vi "mav_crc_read.vi"(11 "byte_array_in":u8[](array[numeric])=[9, 19, 1, 1, 0, 0, 0, 0, 0, 2, 3, 81, 4, 3]) -> (3 "CRC":bool)   [LabVIEW 2023]
panel:
  out "Incoming Checksum":u16
  out "Calculated Checksum":u16
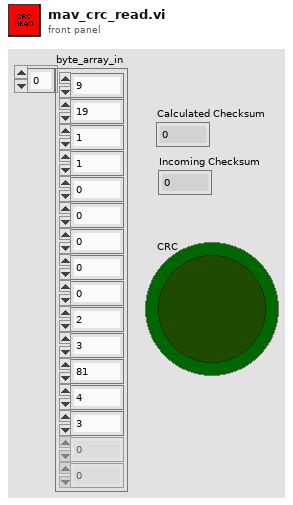
[diagram p1: front panel]
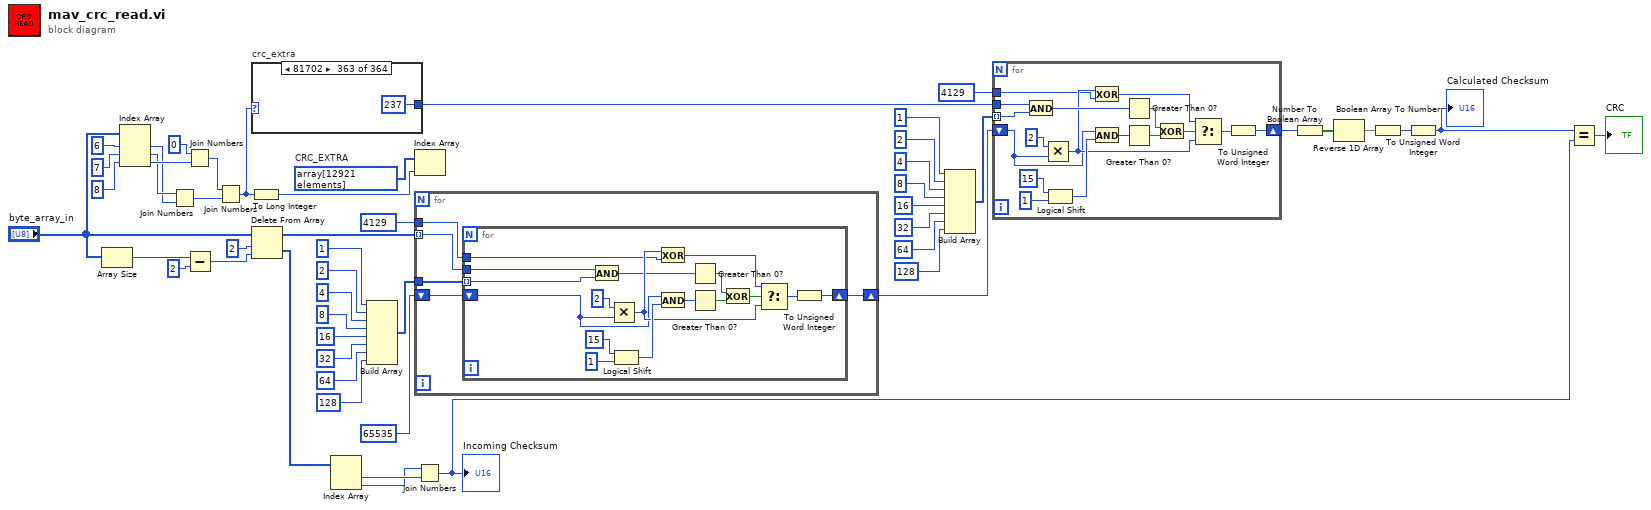
[diagram p0: block diagram]
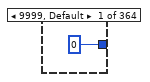
[diagram p2: hidden frame]
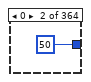
[diagram p3: hidden frame]
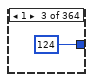
[diagram p4: hidden frame]
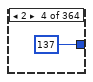
[diagram p5: hidden frame]
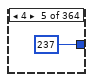
[diagram p6: hidden frame]
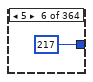
[diagram p7: hidden frame]
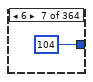
[diagram p8: hidden frame]
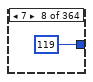
[diagram p9: hidden frame]
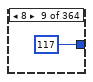
[diagram p10: hidden frame]
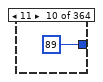
[diagram p11: hidden frame]
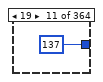
[diagram p12: hidden frame]
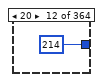
[diagram p13: hidden frame]
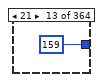
[diagram p14: hidden frame]
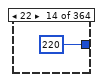
[diagram p15: hidden frame]
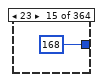
[diagram p16: hidden frame]
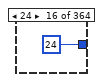
[diagram p17: hidden frame]
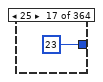
[diagram p18: hidden frame]
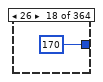
[diagram p19: hidden frame]
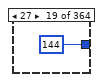
[diagram p20: hidden frame]
diagram:
  w25 = u8[] array[12921 elements]  # CRC_EXTRA
  n1 = Array Size(array="byte_array_in") -> (size(s)=w24:i32)
  n2 = Index Array(array="byte_array_in", index #1=6 ("index"), index #2=7 ("index"), index #3=8 ("index")) -> (element #1=w9:u8, element #2=w10:u8, element #3=w11:u8)
  n3 = Join Numbers(hi=w10, lo=w9) -> ((hi.lo)=w13:u16)
  n4 = Join Numbers(hi=u8 0, lo=w11) -> ((hi.lo)=w12:u16)
  n5 = Subtract(x=w24, y=2) -> (x-y=w23:i32)
  n6 = Join Numbers(hi=w12, lo=w13) -> ((hi.lo)=w3:u32)
  n7 = To Long Integer(number=w3) -> (32bit integer=w14:i32)
  n8 = case "crc_extra" shown="81702" w3 {
    tunnel: [u8 0 ("unsigned byte array 2") u8 50 ("unsigned byte array 2") u8 124 ("unsigned byte array 2") u8 137 ("unsigned byte array 2") u8 237 ("unsigned byte array 2") u8 217 ("unsigned byte array 2") u8 104 ("unsigned byte array 2") u8 119 ("unsigned byte array 2") u8 117 ("unsigned byte array 2") u8 89 ("unsigned byte array 2") u8 137 ("unsigned byte array 2") u8 214 ("unsigned byte array 2") u8 159 ("unsigned byte array 2") u8 220 ("unsigned byte array 2") u8 168 ("unsigned byte array 2") u8 24 ("unsigned byte array 2") u8 23 ("unsigned byte array 2") u8 170 ("unsigned byte array 2") u8 144 ("unsigned byte array 2") u8 67 ("unsigned byte array 2") u8 115 ("unsigned byte array 2") u8 39 ("unsigned byte array 2") u8 246 ("unsigned byte array 2") u8 185 ("unsigned byte array 2") u8 104 ("unsigned byte array 2") u8 237 ("unsigned byte array 2") u8 244 ("unsigned byte array 2") u8 222 ("unsigned byte array 2") u8 212 ("unsigned byte array 2") u8 9 ("unsigned byte array 2") u8 254 ("unsigned byte array 2") u8 230 ("unsigned byte array 2") u8 28 ("unsigned byte array 2") u8 28 ("unsigned byte array 2") u8 132 ("unsigned byte array 2") u8 221 ("unsigned byte array 2") u8 232 ("unsigned byte array 2") u8 11 ("unsigned byte array 2") u8 153 ("unsigned byte array 2") u8 41 ("unsigned byte array 2") u8 39 ("unsigned byte array 2") u8 78 ("unsigned byte array 2") u8 196 ("unsigned byte array 2") u8 15 ("unsigned byte array 2") u8 3 ("unsigned byte array 2") u8 167 ("unsigned byte array 2") u8 183 ("unsigned byte array 2") u8 119 ("unsigned byte array 2") u8 191 ("unsigned byte array 2") u8 118 ("unsigned byte array 2") u8 148 ("unsigned byte array 2") u8 21 ("unsigned byte array 2") u8 243 ("unsigned byte array 2") u8 124 ("unsigned byte array 2") u8 38 ("unsigned byte array 2") u8 20 ("unsigned byte array 2") u8 158 ("unsigned byte array 2") u8 152 ("unsigned byte array 2") u8 143 ("unsigned byte array 2") u8 14 ("unsigned byte array 2") u8 106 ("unsigned byte array 2") u8 49 ("unsigned byte array 2") u8 22 ("unsigned byte array 2") u8 143 ("unsigned byte array 2") u8 140 ("unsigned byte array 2") u8 5 ("unsigned byte array 2") u8 150 ("unsigned byte array 2") u8 231 ("unsigned byte array 2") u8 183 ("unsigned byte array 2") u8 63 ("unsigned byte array 2") u8 54 ("unsigned byte array 2") u8 47 ("unsigned byte array 2") u8 175 ("unsigned byte array 2") u8 102 ("unsigned byte array 2") u8 158 ("unsigned byte array 2") u8 208 ("unsigned byte array 2") u8 56 ("unsigned byte array 2") u8 93 ("unsigned byte array 2") u8 138 ("unsigned byte array 2") u8 108 ("unsigned byte array 2") u8 32 ("unsigned byte array 2") u8 185 ("unsigned byte array 2") u8 84 ("unsigned byte array 2") u8 34 ("unsigned byte array 2") u8 174 ("unsigned byte array 2") u8 124 ("unsigned byte array 2") u8 237 ("unsigned byte array 2") u8 4 ("unsigned byte array 2") u8 76 ("unsigned byte array 2") u8 128 ("unsigned byte array 2") u8 56 ("unsigned byte array 2") u8 116 ("unsigned byte array 2") u8 134 ("unsigned byte array 2") u8 237 ("unsigned byte array 2") u8 203 ("unsigned byte array 2") u8 250 ("unsigned byte array 2") u8 87 ("unsigned byte array 2") u8 203 ("unsigned byte array 2") u8 220 ("unsigned byte array 2") u8 25 ("unsigned byte array 2") u8 226 ("unsigned byte array 2") u8 46 ("unsigned byte array 2") u8 29 ("unsigned byte array 2") u8 223 ("unsigned byte array 2") u8 85 ("unsigned byte array 2") u8 6 ("unsigned byte array 2") u8 229 ("unsigned byte array 2") u8 203 ("unsigned byte array 2") u8 1 ("unsigned byte array 2") u8 195 ("unsigned byte array 2") u8 109 ("unsigned byte array 2") u8 168 ("unsigned byte array 2") u8 181 ("unsigned byte array 2") u8 47 ("unsigned byte array 2") u8 72 ("unsigned byte array 2") u8 131 ("unsigned byte array 2") u8 127 ("unsigned byte array 2") u8 103 ("unsigned byte array 2") u8 154 ("unsigned byte array 2") u8 178 ("unsigned byte array 2") u8 200 ("unsigned byte array 2") u8 134 ("unsigned byte array 2") u8 219 ("unsigned byte array 2") u8 208 ("unsigned byte array 2") u8 188 ("unsigned byte array 2") u8 84 ("unsigned byte array 2") u8 22 ("unsigned byte array 2") u8 19 ("unsigned byte array 2") u8 21 ("unsigned byte array 2") u8 134 ("unsigned byte array 2") u8 78 ("unsigned byte array 2") u8 68 ("unsigned byte array 2") u8 189 ("unsigned byte array 2") u8 127 ("unsigned byte array 2") u8 154 ("unsigned byte array 2") u8 21 ("unsigned byte array 2") u8 21 ("unsigned byte array 2") u8 144 ("unsigned byte array 2") u8 1 ("unsigned byte array 2") u8 234 ("unsigned byte array 2") u8 73 ("unsigned byte array 2") u8 181 ("unsigned byte array 2") u8 22 ("unsigned byte array 2") u8 83 ("unsigned byte array 2") u8 167 ("unsigned byte array 2") u8 138 ("unsigned byte array 2") u8 234 ("unsigned byte array 2") u8 240 ("unsigned byte array 2") u8 47 ("unsigned byte array 2") u8 189 ("unsigned byte array 2") u8 52 ("unsigned byte array 2") u8 174 ("unsigned byte array 2") u8 229 ("unsigned byte array 2") u8 85 ("unsigned byte array 2") u8 159 ("unsigned byte array 2") u8 186 ("unsigned byte array 2") u8 72 ("unsigned byte array 2") u8 92 ("unsigned byte array 2") u8 36 ("unsigned byte array 2") u8 71 ("unsigned byte array 2") u8 98 ("unsigned byte array 2") u8 120 ("unsigned byte array 2") u8 134 ("unsigned byte array 2") u8 205 ("unsigned byte array 2") u8 69 ("unsigned byte array 2") u8 101 ("unsigned byte array 2") u8 50 ("unsigned byte array 2") u8 202 ("unsigned byte array 2") u8 17 ("unsigned byte array 2") u8 162 ("unsigned byte array 2") u8 34 ("unsigned byte array 2") u8 71 ("unsigned byte array 2") u8 15 ("unsigned byte array 2") u8 119 ("unsigned byte array 2") u8 102 ("unsigned byte array 2") u8 208 ("unsigned byte array 2") u8 207 ("unsigned byte array 2") u8 163 ("unsigned byte array 2") u8 105 ("unsigned byte array 2") u8 151 ("unsigned byte array 2") u8 35 ("unsigned byte array 2") u8 150 ("unsigned byte array 2") u8 179 ("unsigned byte array 2") u8 90 ("unsigned byte array 2") u8 104 ("unsigned byte array 2") u8 85 ("unsigned byte array 2") u8 95 ("unsigned byte array 2") u8 130 ("unsigned byte array 2") u8 184 ("unsigned byte array 2") u8 81 ("unsigned byte array 2") u8 8 ("unsigned byte array 2") u8 204 ("unsigned byte array 2") u8 49 ("unsigned byte array 2") u8 170 ("unsigned byte array 2") u8 44 ("unsigned byte array 2") u8 83 ("unsigned byte array 2") u8 46 ("unsigned byte array 2") u8 71 ("unsigned byte array 2") u8 131 ("unsigned byte array 2") u8 187 ("unsigned byte array 2") u8 92 ("unsigned byte array 2") u8 146 ("unsigned byte array 2") u8 179 ("unsigned byte array 2") u8 12 ("unsigned byte array 2") u8 133 ("unsigned byte array 2") u8 49 ("unsigned byte array 2") u8 26 ("unsigned byte array 2") u8 193 ("unsigned byte array 2") u8 35 ("unsigned byte array 2") u8 14 ("unsigned byte array 2") u8 109 ("unsigned byte array 2") u8 59 ("unsigned byte array 2") u8 22 ("unsigned byte array 2") u8 126 ("unsigned byte array 2") u8 18 ("unsigned byte array 2") u8 70 ("unsigned byte array 2") u8 48 ("unsigned byte array 2") u8 123 ("unsigned byte array 2") u8 74 ("unsigned byte array 2") u8 99 ("unsigned byte array 2") u8 137 ("unsigned byte array 2") u8 210 ("unsigned byte array 2") u8 1 ("unsigned byte array 2") u8 20 ("unsigned byte array 2") u8 251 ("unsigned byte array 2") u8 10 ("unsigned byte array 2") u8 234 ("unsigned byte array 2") u8 237 ("unsigned byte array 2") u8 19 ("unsigned byte array 2") u8 217 ("unsigned byte array 2") u8 243 ("unsigned byte array 2") u8 28 ("unsigned byte array 2") u8 95 ("unsigned byte array 2") u8 243 ("unsigned byte array 2") u8 88 ("unsigned byte array 2") u8 243 ("unsigned byte array 2") u8 78 ("unsigned byte array 2") u8 132 ("unsigned byte array 2") u8 23 ("unsigned byte array 2") u8 91 ("unsigned byte array 2") u8 236 ("unsigned byte array 2") u8 231 ("unsigned byte array 2") u8 72 ("unsigned byte array 2") u8 225 ("unsigned byte array 2") u8 245 ("unsigned byte array 2") u8 199 ("unsigned byte array 2") u8 99 ("unsigned byte array 2") u8 232 ("unsigned byte array 2") u8 210 ("unsigned byte array 2") u8 6 ("unsigned byte array 2") u8 11 ("unsigned byte array 2") u8 93 ("unsigned byte array 2") u8 151 ("unsigned byte array 2") u8 26 ("unsigned byte array 2") u8 117 ("unsigned byte array 2") u8 251 ("unsigned byte array 2") u8 232 ("unsigned byte array 2") u8 147 ("unsigned byte array 2") u8 132 ("unsigned byte array 2") u8 4 ("unsigned byte array 2") u8 8 ("unsigned byte array 2") u8 156 ("unsigned byte array 2") u8 0 ("unsigned byte array 2") u8 50 ("unsigned byte array 2") u8 182 ("unsigned byte array 2") u8 110 ("unsigned byte array 2") u8 183 ("unsigned byte array 2") u8 160 ("unsigned byte array 2") u8 106 ("unsigned byte array 2") u8 33 ("unsigned byte array 2") u8 77 ("unsigned byte array 2") u8 109 ("unsigned byte array 2") u8 161 ("unsigned byte array 2") u8 20 ("unsigned byte array 2") u8 134 ("unsigned byte array 2") u8 193 ("unsigned byte array 2") u8 30 ("unsigned byte array 2") u8 66 ("unsigned byte array 2") u8 245 ("unsigned byte array 2") u8 28 ("unsigned byte array 2") u8 218 ("unsigned byte array 2") u8 231 ("unsigned byte array 2") u8 172 ("unsigned byte array 2") u8 251 ("unsigned byte array 2") u8 97 ("unsigned byte array 2") u8 64 ("unsigned byte array 2") u8 234 ("unsigned byte array 2") u8 144 ("unsigned byte array 2") u8 155 ("unsigned byte array 2") u8 20 ("unsigned byte array 2") u8 54 ("unsigned byte array 2") u8 222 ("unsigned byte array 2") u8 200 ("unsigned byte array 2") u8 23 ("unsigned byte array 2") u8 149 ("unsigned byte array 2") u8 113 ("unsigned byte array 2") u8 117 ("unsigned byte array 2") u8 209 ("unsigned byte array 2") u8 186 ("unsigned byte array 2") u8 4 ("unsigned byte array 2") u8 134 ("unsigned byte array 2") u8 15 ("unsigned byte array 2") u8 234 ("unsigned byte array 2") u8 64 ("unsigned byte array 2") u8 46 ("unsigned byte array 2") u8 106 ("unsigned byte array 2") u8 205 ("unsigned byte array 2") u8 144 ("unsigned byte array 2") u8 133 ("unsigned byte array 2") u8 85 ("unsigned byte array 2") u8 195 ("unsigned byte array 2") u8 79 ("unsigned byte array 2") u8 128 ("unsigned byte array 2") u8 177 ("unsigned byte array 2") u8 130 ("unsigned byte array 2") u8 47 ("unsigned byte array 2") u8 142 ("unsigned byte array 2") u8 114 ("unsigned byte array 2") u8 254 ("unsigned byte array 2") u8 140 ("unsigned byte array 2") u8 249 ("unsigned byte array 2") u8 77 ("unsigned byte array 2") u8 49 ("unsigned byte array 2") u8 94 ("unsigned byte array 2") u8 139 ("unsigned byte array 2") u8 7 ("unsigned byte array 2") u8 20 ("unsigned byte array 2") u8 103 ("unsigned byte array 2") u8 26 ("unsigned byte array 2") u8 72 ("unsigned byte array 2") u8 19 ("unsigned byte array 2") u8 89 ("unsigned byte array 2") u8 27 ("unsigned byte array 2") u8 14 ("unsigned byte array 2") u8 187 ("unsigned byte array 2") u8 106 ("unsigned byte array 2") u8 227 ("unsigned byte array 2") u8 239 ("unsigned byte array 2") u8 246 ("unsigned byte array 2") u8 181 ("unsigned byte array 2") u8 62 ("unsigned byte array 2") u8 240 ("unsigned byte array 2") u8 152 ("unsigned byte array 2") u8 13 ("unsigned byte array 2") u8 239 ("unsigned byte array 2") u8 24 ("unsigned byte array 2") u8 166 ("unsigned byte array 2") u8 39 ("unsigned byte array 2") u8 145 ("unsigned byte array 2") u8 208 ("unsigned byte array 2") u8 183 ("unsigned byte array 2") u8 99 ("unsigned byte array 2") u8 129 ("unsigned byte array 2") u8 134 ("unsigned byte array 2") u8 202 ("unsigned byte array 2") u8 156 ("unsigned byte array 2") u8 191 ("unsigned byte array 2") u8 220 ("unsigned byte array 2") u8 245 ("unsigned byte array 2") u8 101 ("unsigned byte array 2") u8 45 ("unsigned byte array 2") u8 246 ("unsigned byte array 2") u8 237 ("unsigned byte array 2") u8 216 ("unsigned byte array 2")] -> w1
    frame 9999, Default {
    }
    frame 0 {
    }
    frame 1 {
    }
    frame 2 {
    }
    frame 4 {
    }
    frame 5 {
    }
    frame 6 {
    }
    frame 7 {
    }
    frame 8 {
    }
    frame 11 {
    }
    frame 19 {
    }
    frame 20 {
    }
    frame 21 {
    }
    frame 22 {
    }
    frame 23 {
    }
    frame 24 {
    }
    frame 25 {
    }
    frame 26 {
    }
    frame 27 {
    }
    frame 28 {
    }
    frame 29 {
    }
    frame 30 {
    }
    frame 31 {
    }
    frame 32 {
    }
    frame 33 {
    }
    frame 34 {
    }
    frame 35 {
    }
    frame 36 {
    }
    frame 37 {
    }
    frame 38 {
    }
    frame 39 {
    }
    frame 40 {
    }
    frame 41 {
    }
    frame 42 {
    }
    frame 43 {
    }
    frame 44 {
    }
    frame 45 {
    }
    frame 46 {
    }
    frame 47 {
    }
    frame 48 {
    }
    frame 49 {
    }
    frame 50 {
    }
    frame 51 {
    }
    frame 54 {
    }
    frame 55 {
    }
    frame 61 {
    }
    frame 62 {
    }
    frame 63 {
    }
    frame 64 {
    }
    frame 65 {
    }
    frame 66 {
    }
    frame 67 {
    }
    frame 69 {
    }
    frame 70 {
    }
    frame 73 {
    }
    frame 74 {
    }
    frame 75 {
    }
    frame 76 {
    }
    frame 77 {
    }
    frame 80 {
    }
    frame 81 {
    }
    frame 82 {
    }
    frame 83 {
    }
    frame 84 {
    }
    frame 85 {
    }
    frame 86 {
    }
    frame 87 {
    }
    frame 89 {
    }
    frame 90 {
    }
    frame 91 {
    }
    frame 92 {
    }
    frame 93 {
    }
    frame 100 {
    }
    frame 101 {
    }
    frame 102 {
    }
    frame 103 {
    }
    frame 104 {
    }
    frame 105 {
    }
    frame 106 {
    }
    frame 107 {
    }
    frame 108 {
    }
    frame 109 {
    }
    frame 110 {
    }
    frame 111 {
    }
    frame 112 {
    }
    frame 113 {
    }
    frame 114 {
    }
    frame 115 {
    }
    frame 116 {
    }
    frame 117 {
    }
    frame 118 {
    }
    frame 119 {
    }
    frame 120 {
    }
    frame 121 {
    }
    frame 122 {
    }
    frame 123 {
    }
    frame 124 {
    }
    frame 125 {
    }
    frame 126 {
    }
    frame 127 {
    }
    frame 128 {
    }
    frame 129 {
    }
    frame 130 {
    }
    frame 131 {
    }
    frame 132 {
    }
    frame 133 {
    }
    frame 134 {
    }
    frame 135 {
    }
    frame 136 {
    }
    frame 137 {
    }
    frame 138 {
    }
    frame 139 {
    }
    frame 140 {
    }
    frame 141 {
    }
    frame 142 {
    }
    frame 143 {
    }
    frame 144 {
    }
    frame 146 {
    }
    frame 147 {
    }
    frame 148 {
    }
    frame 149 {
    }
    frame 150 {
    }
    frame 151 {
    }
    frame 152 {
    }
    frame 153 {
    }
    frame 154 {
    }
    frame 155 {
    }
    frame 156 {
    }
    frame 157 {
    }
    frame 158 {
    }
    frame 160 {
    }
    frame 161 {
    }
    frame 162 {
    }
    frame 163 {
    }
    frame 164 {
    }
    frame 165 {
    }
    frame 166 {
    }
    frame 167 {
    }
    frame 168 {
    }
    frame 169 {
    }
    frame 170 {
    }
    frame 171 {
    }
    frame 172 {
    }
    frame 173 {
    }
    frame 174 {
    }
    frame 175 {
    }
    frame 176 {
    }
    frame 177 {
    }
    frame 178 {
    }
    frame 179 {
    }
    frame 180 {
    }
    frame 181 {
    }
    frame 182 {
    }
    frame 183 {
    }
    frame 184 {
    }
    frame 185 {
    }
    frame 186 {
    }
    frame 191 {
    }
    frame 192 {
    }
    frame 193 {
    }
    frame 194 {
    }
    frame 195 {
    }
    frame 200 {
    }
    frame 201 {
    }
    frame 214 {
    }
    frame 215 {
    }
    frame 216 {
    }
    frame 217 {
    }
    frame 218 {
    }
    frame 219 {
    }
    frame 220 {
    }
    frame 221 {
    }
    frame 222 {
    }
    frame 223 {
    }
    frame 224 {
    }
    frame 225 {
    }
    frame 226 {
    }
    frame 230 {
    }
    frame 231 {
    }
    frame 232 {
    }
    frame 233 {
    }
    frame 234 {
    }
    frame 235 {
    }
    frame 241 {
    }
    frame 242 {
    }
    frame 243 {
    }
    frame 244 {
    }
    frame 245 {
    }
    frame 246 {
    }
    frame 247 {
    }
    frame 248 {
    }
    frame 249 {
    }
    frame 250 {
    }
    frame 251 {
    }
    frame 252 {
    }
    frame 253 {
    }
    frame 254 {
    }
    frame 256 {
    }
    frame 257 {
    }
    frame 258 {
    }
    frame 259 {
    }
    frame 260 {
    }
    frame 261 {
    }
    frame 262 {
    }
    frame 263 {
    }
    frame 264 {
    }
    frame 265 {
    }
    frame 266 {
    }
    frame 267 {
    }
    frame 268 {
    }
    frame 269 {
    }
    frame 270 {
    }
    frame 271 {
    }
    frame 275 {
    }
    frame 276 {
    }
    frame 280 {
    }
    frame 281 {
    }
    frame 282 {
    }
    frame 283 {
    }
    frame 284 {
    }
    frame 285 {
    }
    frame 286 {
    }
    frame 287 {
    }
    frame 288 {
    }
    frame 290 {
    }
    frame 291 {
    }
    frame 295 {
    }
    frame 298 {
    }
    frame 299 {
    }
    frame 300 {
    }
    frame 301 {
    }
    frame 310 {
    }
    frame 311 {
    }
    frame 320 {
    }
    frame 321 {
    }
    frame 322 {
    }
    frame 323 {
    }
    frame 324 {
    }
    frame 330 {
    }
    frame 331 {
    }
    frame 332 {
    }
    frame 333 {
    }
    frame 334 {
    }
    frame 335 {
    }
    frame 336 {
    }
    frame 339 {
    }
    frame 340 {
    }
    frame 350 {
    }
    frame 354 {
    }
    frame 355 {
    }
    frame 360 {
    }
    frame 361 {
    }
    frame 369 {
    }
    frame 370 {
    }
    frame 373 {
    }
    frame 375 {
    }
    frame 380 {
    }
    frame 385 {
    }
    frame 386 {
    }
    frame 387 {
    }
    frame 388 {
    }
    frame 390 {
    }
    frame 395 {
    }
    frame 396 {
    }
    frame 397 {
    }
    frame 400 {
    }
    frame 401 {
    }
    frame 410 {
    }
    frame 411 {
    }
    frame 412 {
    }
    frame 413 {
    }
    frame 414 {
    }
    frame 415 {
    }
    frame 420 {
    }
    frame 435 {
    }
    frame 436 {
    }
    frame 437 {
    }
    frame 440 {
    }
    frame 510 {
    }
    frame 511 {
    }
    frame 8002 {
    }
    frame 8003 {
    }
    frame 8004 {
    }
    frame 8005 {
    }
    frame 8006 {
    }
    frame 8007 {
    }
    frame 8008 {
    }
    frame 8009 {
    }
    frame 8010 {
    }
    frame 8011 {
    }
    frame 8012 {
    }
    frame 8013 {
    }
    frame 8014 {
    }
    frame 8015 {
    }
    frame 8016 {
    }
    frame 9000 {
    }
    frame 9005 {
    }
    frame 10001 {
    }
    frame 10002 {
    }
    frame 10003 {
    }
    frame 11000 {
    }
    frame 11001 {
    }
    frame 11002 {
    }
    frame 11003 {
    }
    frame 11010 {
    }
    frame 11011 {
    }
    frame 11020 {
    }
    frame 11030 {
    }
    frame 11031 {
    }
    frame 11032 {
    }
    frame 11033 {
    }
    frame 11034 {
    }
    frame 11035 {
    }
    frame 11036 {
    }
    frame 11037 {
    }
    frame 11038 {
    }
    frame 11039 {
    }
    frame 12900 {
    }
    frame 12901 {
    }
    frame 12902 {
    }
    frame 12903 {
    }
    frame 12904 {
    }
    frame 12905 {
    }
    frame 12915 {
    }
    frame 12918 {
    }
    frame 12919 {
    }
    frame 12920 {
    }
    frame 17000 {
    }
    frame 17150 {
    }
    frame 17151 {
    }
    frame 17153 {
    }
    frame 17154 {
    }
    frame 17155 {
    }
    frame 17156 {
    }
    frame 17157 {
    }
    frame 17158 {
    }
    frame 42000 {
    }
    frame 42001 {
    }
    frame 50001 {
    }
    frame 50002 {
    }
    frame 50003 {
    }
    frame 50004 {
    }
    frame 50005 {
    }
    frame 52000 {
    }
    frame 52001 {
    }
    frame 52002 {
    }
    frame 52003 {
    }
    frame 52004 {
    }
    frame 52005 {
    }
    frame 60010 {
    }
    frame 60011 {
    }
    frame 60012 {
    }
    frame 60013 {
    }
    frame 60014 {
    }
    frame 60020 {
    }
    frame 60040 {
    }
    frame 60041 {
    }
    frame 60050 {
    }
    frame 60051 {
    }
    frame 60052 {
    }
    frame 60053 {
    }
    frame 81701 {
    }
    frame 81702 {
    }
    frame 81703 {
    }
  }
  n9 = Delete From Array(array="byte_array_in", length=2 ("y"), index=w23) -> (deleted portion=w21:u8[], array with subset deleted=w20:u8[])
  n10 = Index Array(array=w21) -> (element #1=w16:u8, element #2=w15:u8)  [unwired: 2 in]
  n11 = Build Array(u8 1, u8 2, u8 4, u8 8, u8 16, u8 32, u8 64, u8 128) -> (w42:u8[])
  n12 = Index Array(array=w25, index=w14) -> ()  [unwired: 1 out]
  n13 = for {
    shift-right: [w419] -> w26
    shift-left: u16 65535 -> [w420]
    tunnel: w20 -> [w418] mode=indexing
    tunnel: w42 -> [w417]
    tunnel: u16 4129 -> [w416]
    n14 = for {
      shift-right: [w436] -> w419
      shift-left: w420 -> [w427]
      tunnel: w417 -> [w428] mode=indexing
      tunnel: w418 -> [w423]
      tunnel: w416 -> [w422]
      n15 = And(x=w423, y=w428) -> (x .and. y?=w421:u8)
      n16 = Multiply(x=u16 2, y=w427) -> (x*y=w429:u16)
      n17 = Logical Shift(y=u16 15 ("Numeric"), x=u16 1 ("Numeric 2")) -> (x << y=w431:u16)
      n18 = Exclusive Or(1:w422, 2:w429) -> (0:w437:u16)
      n19 = And(x=w427, y=w431) -> (x .and. y?=w430:u16)
      n20 = Greater Than 0?(x=w421) -> (x > 0?=w434:bool)
      n21 = Greater Than 0?(x=w430) -> (x > 0?=w425:bool)
      n22 = Exclusive Or(1:w425, 2:w434) -> (0:w424:bool)
      n23 = Select(t=w437, s=w424, f=w429) -> (s? t:f=w435:u16)
      n24 = To Unsigned Word Integer(number=w435) -> (unsigned 16bit integer=w436:u16)
    }
  }
  n25 = Join Numbers(hi=w15, lo=w16) -> ((hi.lo)=w18:u16)
  "Incoming Checksum" <- w18
  n26 = Build Array(u8 1, u8 2, u8 4, u8 8, u8 16, u8 32, u8 64, u8 128) -> (w36:u8[])
  n27 = for {
    shift-right: [w453] -> w27
    shift-left: w26 -> [w443]
    tunnel: w36 -> [w444] mode=indexing
    tunnel: w1 -> [w439]
    tunnel: u16 4129 -> [w438]
    n28 = And(x=w439, y=w444) -> (x .and. y?=w451:u8)
    n29 = Multiply(x=u16 2, y=w443) -> (x*y=w445:u16)
    n30 = Logical Shift(y=u16 15, x=u16 1) -> (x << y=w447:u16)
    n31 = Exclusive Or(1:w438, 2:w445) -> (0:w454:u16)
    n32 = And(x=w443, y=w447) -> (x .and. y?=w446:u16)
    n33 = Greater Than 0?(x=w451) -> (x > 0?=w450:bool)
    n34 = Greater Than 0?(x=w446) -> (x > 0?=w441:bool)
    n35 = Exclusive Or(1:w441, 2:w450) -> (0:w440:bool)
    n36 = Select(t=w454, s=w440, f=w445) -> (s? t:f=w452:u16)
    n37 = To Unsigned Word Integer(number=w452) -> (unsigned 16bit integer=w453:u16)
  }
  n38 = Number To Boolean Array(number=w27) -> (Boolean array=w41:bool[])
  n39 = Reverse 1D Array(array=w41) -> (reversed array=w40:bool[])
  n40 = Boolean Array To Number(Boolean array=w40) -> (number=w39:u32)
  n41 = To Unsigned Word Integer(number=w39) -> (unsigned 16bit integer=w19:u16)
  "Calculated Checksum" <- w19
  n42 = Equal?(x=w19, y=w18) -> (x = y?=→"CRC":bool)
